vi "自校准.vi"   [LabVIEW 2012]
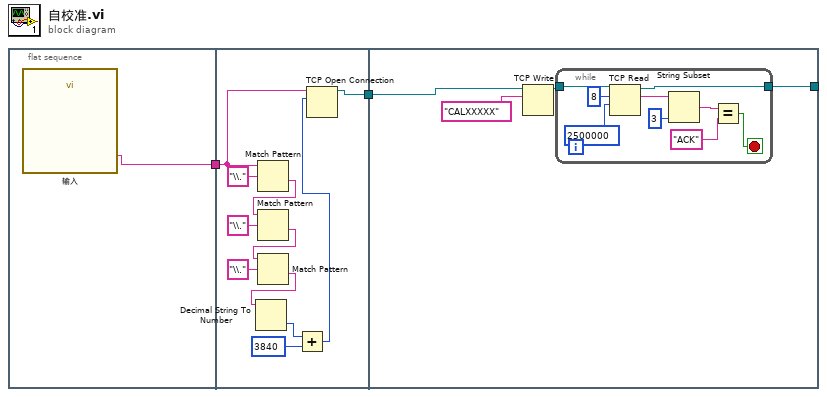
[diagram p0: block diagram]
diagram:
  n1 = flat-sequence {
    tunnel: [w3] -> w2
    tunnel: [w14] -> w1
    tunnel: w2 -> [w8]
    tunnel: w1 -> [w18]
    tunnel: [w16] -> _
    frame #0 {
      n2 = call "输入"() -> ("IP地址"=w3:string)  [unwired: 17 in, 2 out]
    }
    frame #1 {
      n3 = Match Pattern(string=w8, regular expression="\\." ("正则表达式")) -> (after substring=w10:string)  [unwired: 1 in, 3 out]
      n4 = Match Pattern(string=w10, regular expression="\\." ("正则表达式")) -> (after substring=w9:string)  [unwired: 1 in, 3 out]
      n5 = Match Pattern(string=w9, regular expression="\\." ("正则表达式")) -> (after substring=w7:string)  [unwired: 1 in, 3 out]
      n6 = Decimal String To Number(string=w7) -> (number=w6:i32)  [unwired: 2 in, 1 out]
      n7 = Add(x=w6, y=3840) -> (x+y=w4:i32)
      n8 = TCP Open Connection(address=w8, remote port or service name=w4) -> (connection ID=w14:refnum<k5>)  [unwired: 3 in, 1 out]
    }
    frame #2 {
      n9 = TCP Write(connection ID=w18, data in="CALXXXXX" ("数据输入")) -> (connection ID out=w17:refnum<k5>)  [unwired: 2 in, 2 out]
      n10 = while {
        tunnel: w17 -> [w27]
        tunnel: [w21] -> w16
        stop <- w22 stop-if-true
        n11 = TCP Read(connection ID=w27, bytes to read=8 ("读取的字节"), 9:2500000 ("超时毫秒(25000)")) -> (connection ID out=w21:refnum<k5>, data out=w25:string)  [unwired: 2 in, 1 out]
        n12 = String Subset(string=w25, length (rest)=3 ("偏移量(0)")) -> (substring=w24:string)  [unwired: 1 in]
        n13 = Equal?(x=w24, y="ACK") -> (x = y?=w22:bool)
      }
    }
  }
